vi "Main.vi"(8 "error in":errorcluster, 11 "Workers in":refnum<class "Workers.lvclass">) -> (0 "error out":errorcluster, 3 "Workers out":refnum<class "Workers.lvclass">)   [LabVIEW 2025, in "Workers.lvclass"]
doc: "The <b>Queued Message Handler</b> of the Worker that owns this VI."
uses:
  Workers.lvclass
  C:/Program Files (x86)/National Instruments/LabVIEW 2025/vi.lib/addons/_Workers/Library/Classes/Worker/Worker.lvclass
  Initialization Data.ctl
  Response Cases.ctl
  Workers.lvclass/Workers.ctl
  AnotherWorkers/AnotherWorkers.lvclass
  rql_PressGetDateTime.ctl
  rql_PressGenerateRandomNum.ctl
  rql_PressReturnRandomNum.ctl
  rql_PressReturnPasswordKey.ctl
  <vilib>/addons/_Workers/Library/Classes/Message Queue/Message Queue.lvclass
  <vilib>/addons/_Workers/Library/Classes/Worker/Worker.lvclass
  C:/Program Files (x86)/National Instruments/LabVIEW 2025/vi.lib/addons/_Workers/Library/Classes/Workers Object/Workers Object.lvclass
  C:/Users/chrismadlax/Desktop/LVSampleCode/WorkersUML/Workers/Workers/Workers.lvclass
  AnotherWorkers/rqp_GeneratePasswordKey.ctl
  C:/Users/chrismadlax/Desktop/LVSampleCode/WorkersUML/Workers/AnotherWorkers/AnotherWorkers.lvclass
panel:
  out "String 2":string
  in  "CallAnotherWorker:ReturnPasswordKEY":bool
  out "String":string
  in  "CallAnotherWorker:ReturnRandomNum":bool
  in  "CallAnotherWorker:GenerateRandomNum":bool
  in  "GetDateTime":bool
  # "Workers"
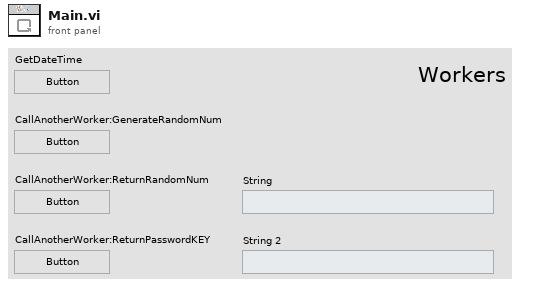
[diagram p1: front panel]
types:
  T1 = typedef "Workers.lvclass/Initialization Data.ctl" = cluster{"Response Cases":T2}
  T2 = typedef "Workers.lvclass/Response Cases.ctl" = cluster{"Placeholder - Can be deleted":string}
  T3 = typedef "Workers.lvclass/rql_PressGetDateTime.ctl" = cluster{"String":string}
  T4 = typedef "Workers.lvclass/rql_PressGenerateRandomNum.ctl" = cluster{"String":string}
  T5 = typedef "Workers.lvclass/rql_PressReturnRandomNum.ctl" = cluster{"String":string}
  T6 = typedef "AnotherWorkers.lvclass/rqp_GeneratePasswordKey.ctl" = cluster{"String":string}
  T7 = typedef "Workers.lvclass/rql_PressReturnPasswordKey.ctl" = cluster{"String":string}
  T8 = typedef "AnotherWorkers.lvclass/rwr_ReturnRandomNumber Reply.ctl" = cluster{"String":string}
  T9 = typedef "Workers.lvlib/Case Label.ctl" = string
  T10 = typedef "AnotherWorkers.lvclass/rsp_ReturnPasswordKey.ctl" = cluster{"String":string}
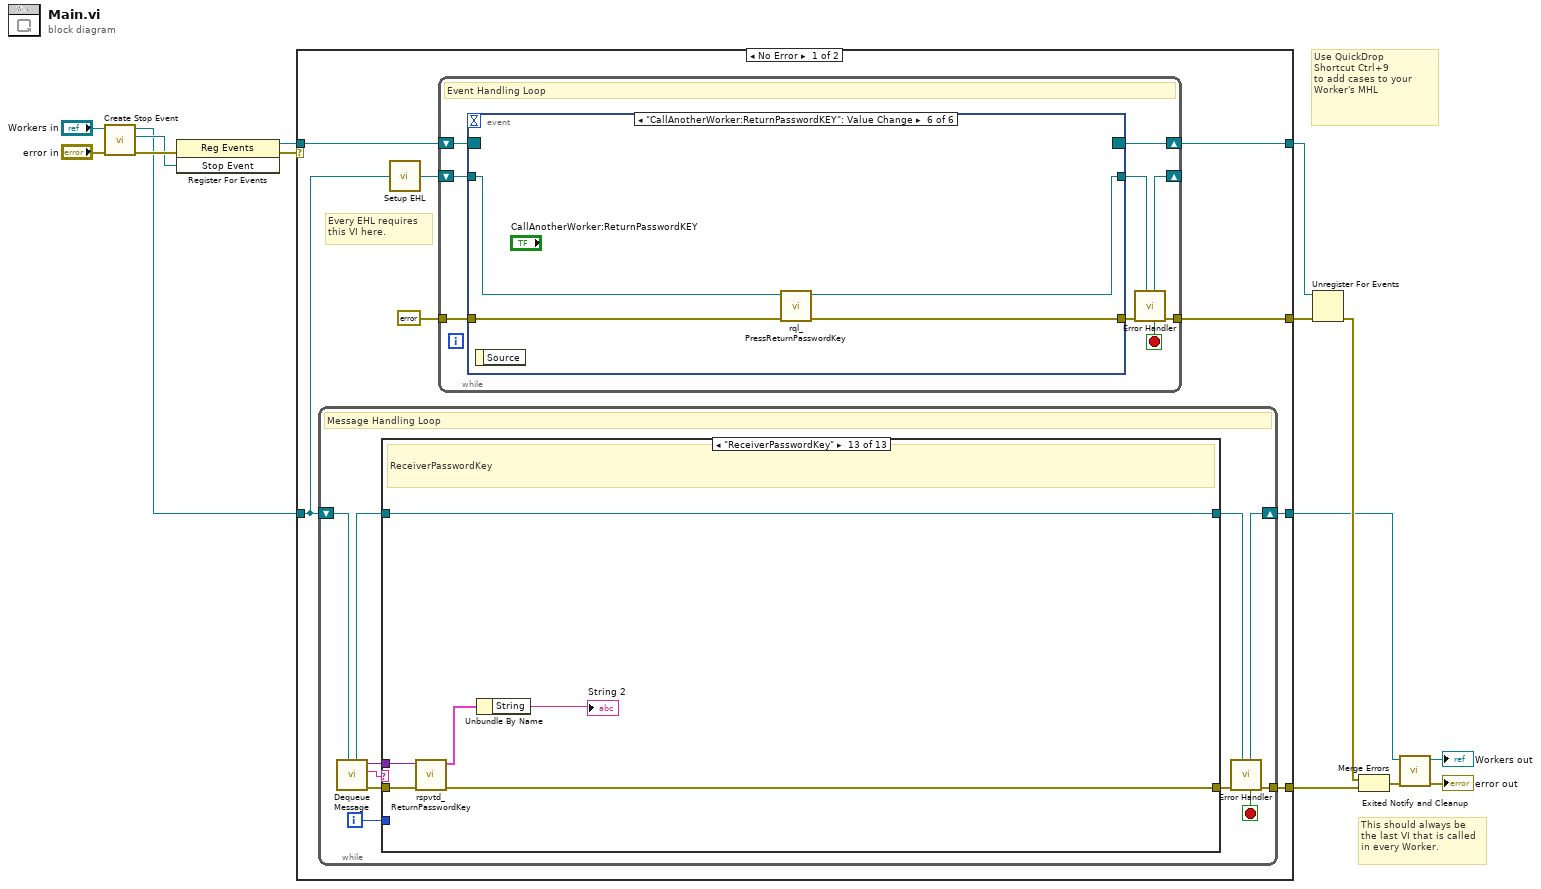
[diagram p0: block diagram]
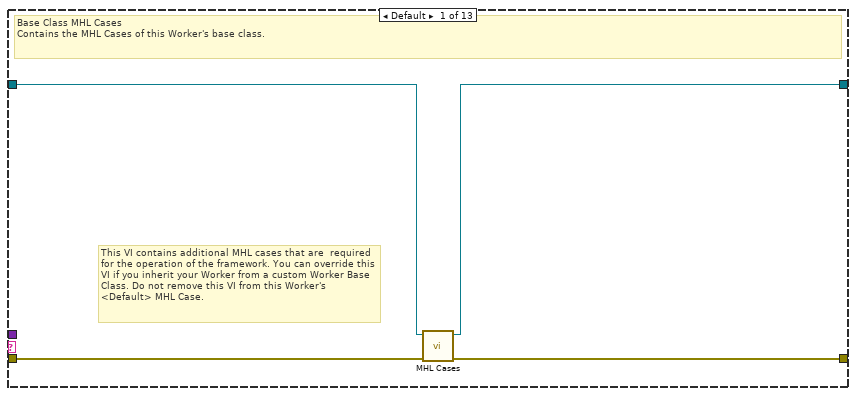
[diagram p2: hidden frame]
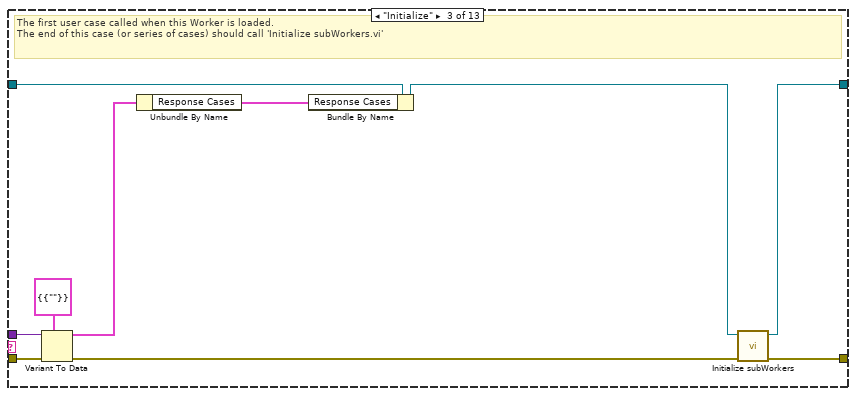
[diagram p4: hidden frame]
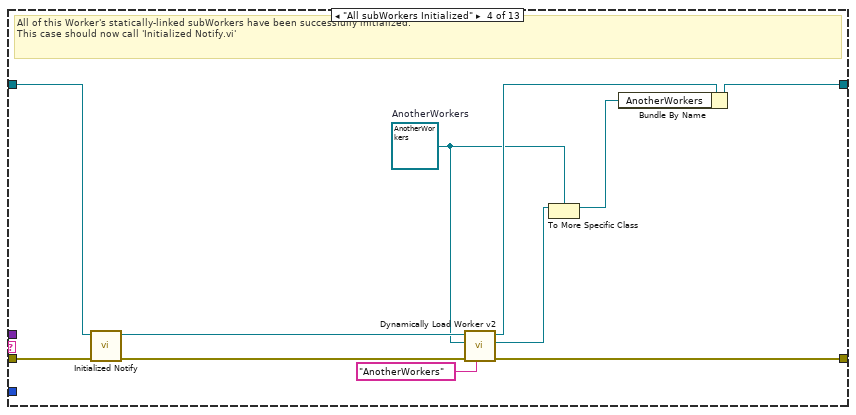
[diagram p5: hidden frame]
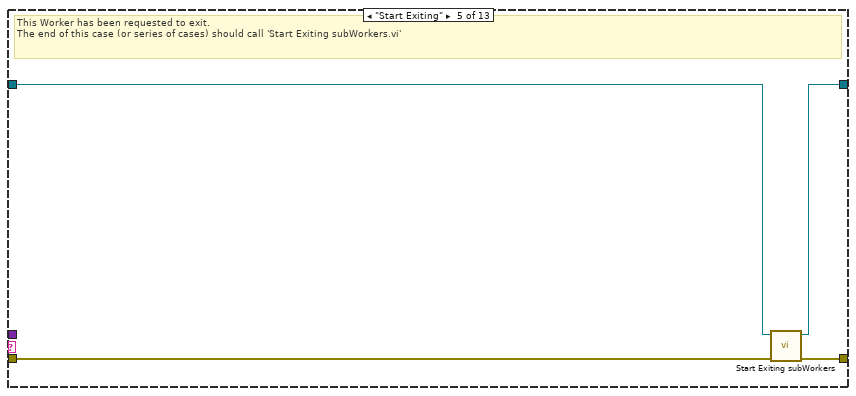
[diagram p6: hidden frame]
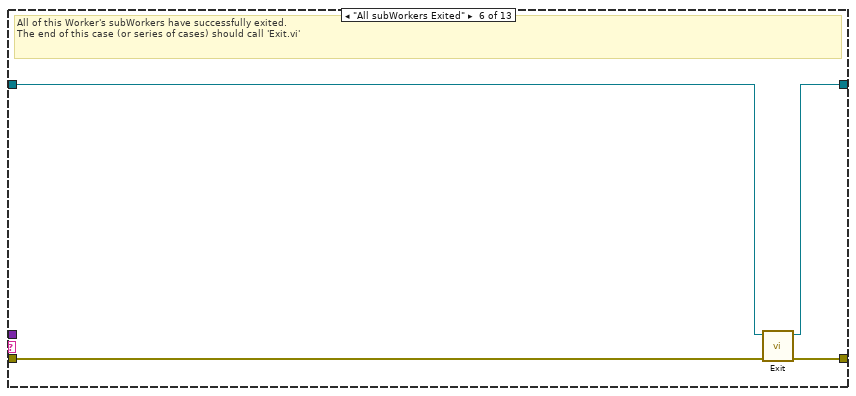
[diagram p7: hidden frame]
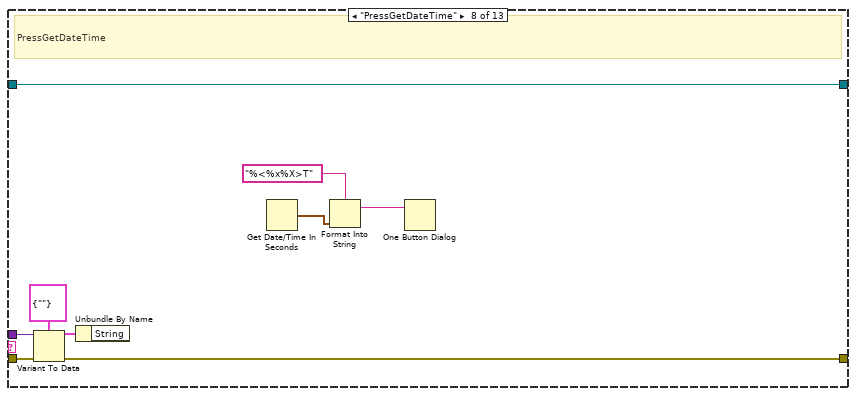
[diagram p9: hidden frame]
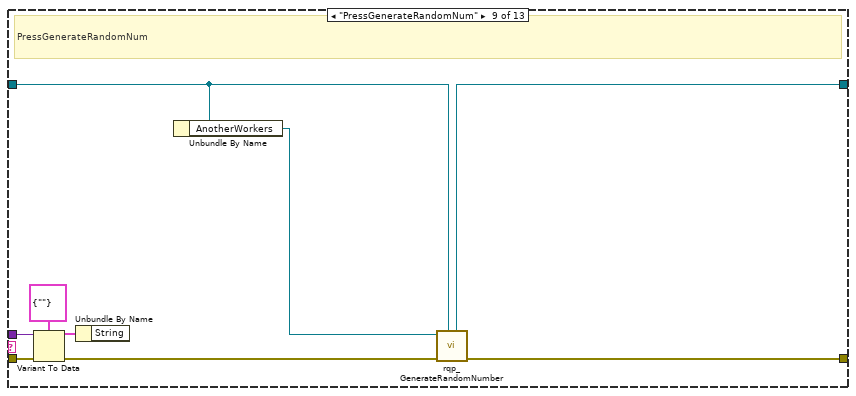
[diagram p10: hidden frame]
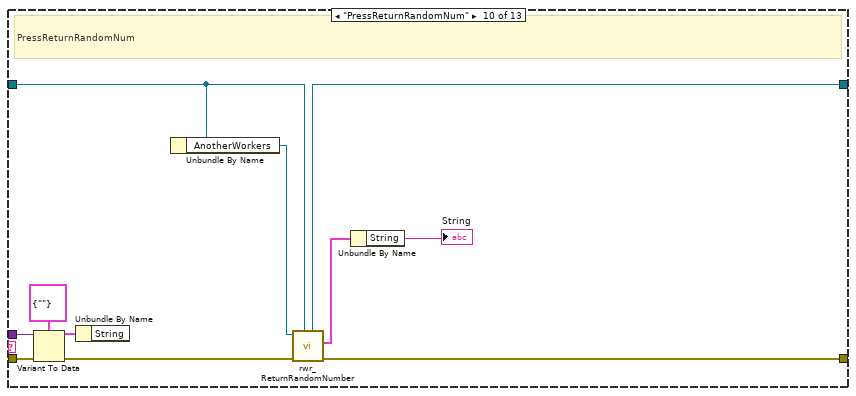
[diagram p11: hidden frame]
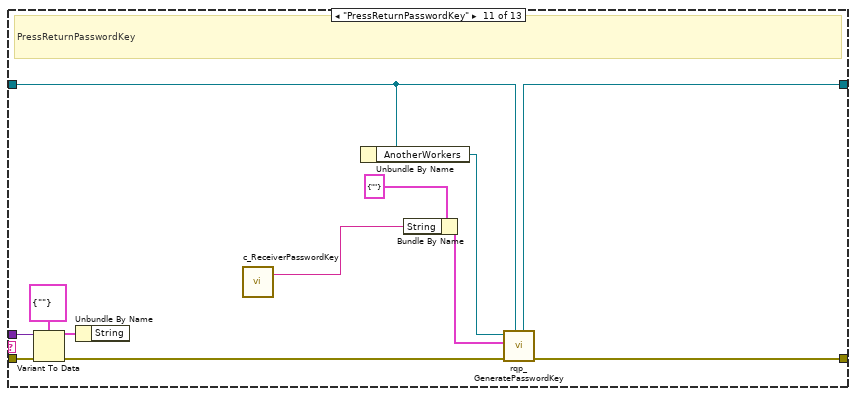
[diagram p12: hidden frame]
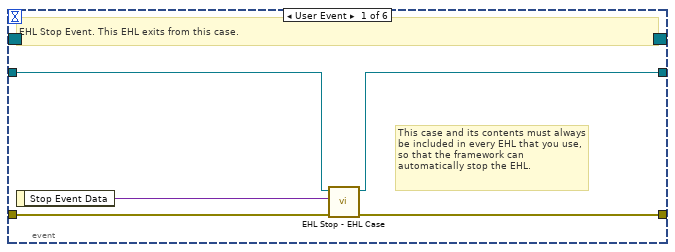
[diagram p14: hidden frame]
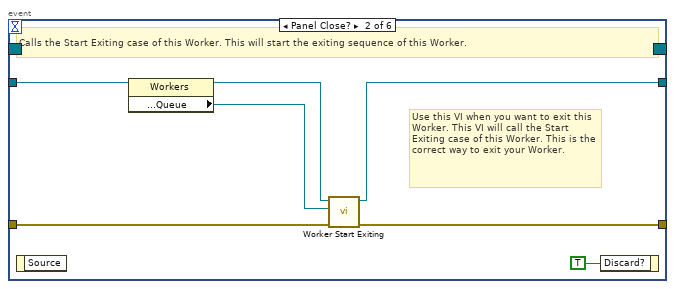
[diagram p15: hidden frame]
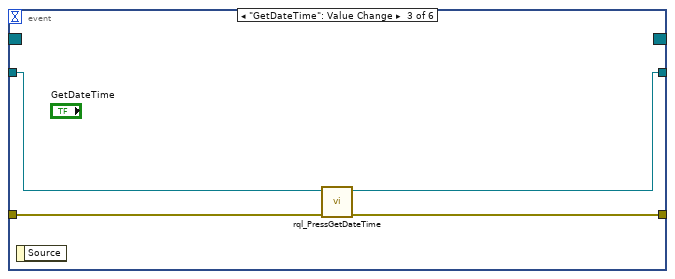
[diagram p16: hidden frame]
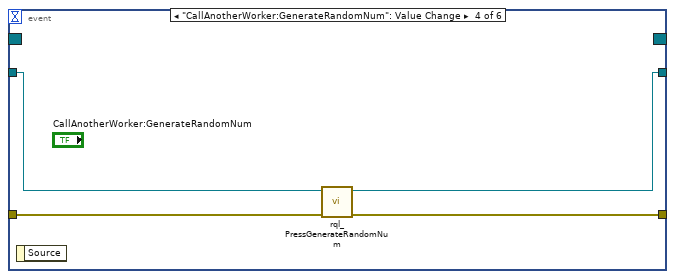
[diagram p17: hidden frame]
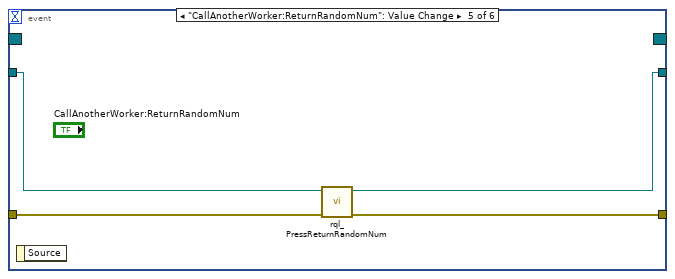
[diagram p18: hidden frame]
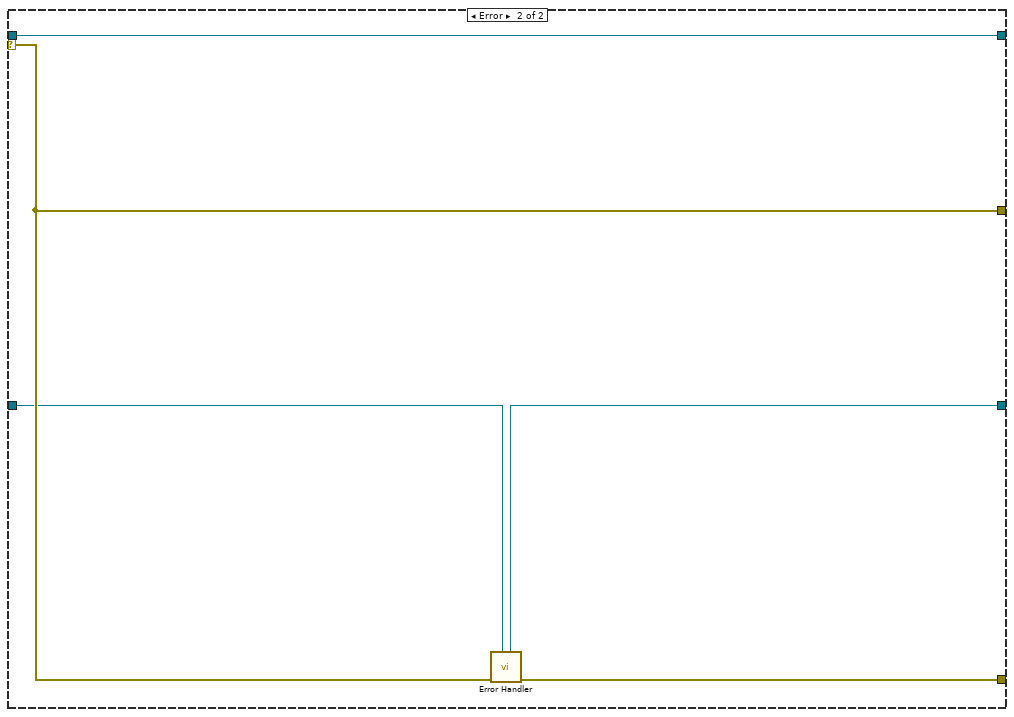
[diagram p19: hidden frame]
diagram:
  # "Use QuickDrop\nShortcut Ctrl+9\nto add cases to your\nWorker's MHL"
  # "This should always be the last VI that is called in every Worker."
  n1 = call-dynamic "Create Stop Event.vi"("error in"="error in", "Worker"="Workers in") -> ("error out"=w10:errorcluster, "Stop Event"=w7:refnum<user-event>, "Worker out"=w4:refnum<class "Workers.lvclass">)  [unwired: 7 in]
  n2 = register-events(error in=w10, w7) -> (reference out=w9:refnum<event-registration>, error out=w1:errorcluster)  [unwired: 1 in]
  n3 = case shown="No Error" w1 {
    tunnel: w4 -> [w18 w159]
    tunnel: [w16 w160] -> w8
    tunnel: w9 -> [w23 w161]
    tunnel: [w20 w162] -> w14
    tunnel: [w22 w161] -> w13
    tunnel: [w17 w158] -> w11
    selector: w1 -> [_ w162]
    frame No Error {
      # "Every EHL requires\nthis VI here."
      n4 = while {
        shift-right: [w32] -> w17
        shift-left: w18 -> [w34]
        tunnel: [w33] -> w16
        i -> [w25]
        stop <- w26 stop-if-true
        # "Message Handling Loop"
        n5 = call-dynamic "Dequeue Message.vi"("Worker"=w34) -> ("error out"=w31:errorcluster, "Case out"=w27:string, "Data out"=w24:variant, "Worker out"=w29:refnum<class "Workers.lvclass">)  [unwired: 6 in, 1 out]
        n6 = case "Worker MHL Case Structure (DO NOT CHANGE LABEL NAME)" shown="\"ReceiverPasswordKey\"" w27 {
          tunnel: w31 -> [w38 w39 w48 w60 w62 w69 w71 w79 w89 w100 w112 w114 w120]
          tunnel: [w37 w39 w50 w58 w65 w68 w71 w78 w84 w95 w107 w114 w118] -> w30
          tunnel: w29 -> [w36 w40 w47 w61 w63 w67 w70 w80 w82 w93 w105 w113 w119]
          tunnel: [w35 w40 w49 w54 w64 w66 w70 w80 w83 w94 w106 w113 w119] -> w28
          tunnel: w25 -> [_ _ _ _ _ _ _ _ _ _ _ _ _]
          tunnel: w24 -> [_ _ w45 _ _ _ _ w76 w86 w97 w109 _ w117]
          frame Default {
            # "This VI contains additional MHL cases that are  required for the operation of the framework. You can override this VI if you inherit your Worker from a custom Worker Base Class. Do not remove this VI from this Worker's <Default> MHL Case."
            # "Base Class MHL Cases\nContains the MHL Cases of this Worker's base class."
            n7 = call-dynamic "MHL Cases.vi"("error in"=w38, "Worker in"=w36) -> ("error out"=w37:errorcluster, "Worker out"=w35:refnum<class "Workers.lvclass">)  [unwired: 8 in]
          }
          frame "------------ FRAMEWORK CASES -----------" {
            # "Start of Workers Framework Cases"
          }
          frame "Initialize" {
            # "The first user case called when this Worker is loaded.\nThe end of this case (or series of cases) should call 'Initialize subWorkers.vi'"
            n8 = Variant To Data(error in=w48, type=T1 {"Response Cases"={"Placeholder - Can be deleted"=""}} ("Initialization Data"), Variant=w45) -> (data=w43:T1, error out=w46:errorcluster)
            n9 = Unbundle By Name(w43) -> ("Response Cases"=w42:T2)
            n10 = Bundle By Name(cluster=w47, "Response Cases"=w42) -> (w44:refnum<class "Workers.lvclass">)
            n11 = call-dynamic "Initialize subWorkers.vi"("error in"=w46, "Worker"=w44) -> ("error out"=w50:errorcluster, "dup Worker out"=w49:refnum<class "Workers.lvclass">)  [unwired: 8 in]
          }
          frame "All subWorkers Initialized" {
            w51 = refnum<class "AnotherWorkers.lvclass"> refnum  # AnotherWorkers
            # "All of this Worker's statically-linked subWorkers have been successfully initialized.\nThis case should now call 'Initialized Notify.vi'"
            n12 = call-dynamic "Initialized Notify.vi"("error in"=w60, "Worker"=w61) -> ("error out"=w59:errorcluster, "dup Worker out"=w57:refnum<class "Workers.lvclass">)  [unwired: 8 in]
            n13 = call <vilib>:"Dynamically Load Worker v2.vi"("Worker Alias"="AnotherWorkers", "error in"=w59, "Worker to Dynamically Load"=w51, "Worker"=w57) -> ("error out"=w58:errorcluster, "Dynamically Loaded Worker out"=w52:refnum<class "Worker.lvclass">, "dup Worker out"=w56:refnum<class "Workers.lvclass">)  [unwired: 5 in]
            n14 = To More Specific Class(target class=w51, reference=w52) -> (specific class reference=w53:refnum<class "AnotherWorkers.lvclass">)  [unwired: 1 in, 1 out]
            n15 = Bundle By Name(cluster=w56, "AnotherWorkers"=w53) -> (w54:refnum<class "Workers.lvclass">)
          }
          frame "Start Exiting" {
            # "This Worker has been requested to exit. \nThe end of this case (or series of cases) should call 'Start Exiting subWorkers.vi'"
            n16 = call-dynamic "Start Exiting subWorkers.vi"("error_in"=w62, "Worker"=w63) -> ("error out"=w65:errorcluster, "dup Worker out"=w64:refnum<class "Workers.lvclass">)  [unwired: 8 in]
          }
          frame "All subWorkers Exited" {
            # "All of this Worker's subWorkers have successfully exited. \nThe end of this case (or series of cases) should call 'Exit.vi'"
            n17 = call-dynamic "Exit.vi"("error_in"=w69, "Worker"=w67) -> ("error out"=w68:errorcluster, "dup Worker out"=w66:refnum<class "Workers.lvclass">)  [unwired: 8 in]
          }
          frame "------------- LOCAL API CASES -------------" {
            # "Start of Workers Local API Cases"
          }
          frame "PressGetDateTime" {
            # "PressGetDateTime"
            n18 = Variant To Data(error in=w79, type=T3 {"String"=""} ("Data"), Variant=w76) -> (data=w75:T3, error out=w78:errorcluster)
            n19 = Unbundle By Name(w75) -> ()  [unwired: 1 out]
            n20 = Get Date/Time In Seconds() -> (seconds since 1Jan1904=w74:timestamp)
            n21 = Format Into String(format string="%<%x%X>T", w74) -> (resulting string=w72:string)  [unwired: 2 in, 1 out]
            n22 = One Button Dialog(message=w72) -> ()  [unwired: 1 in, 1 out]
          }
          frame "PressGenerateRandomNum" {
            # "PressGenerateRandomNum"
            n23 = Variant To Data(error in=w89, type=T4 {"String"=""} ("Data"), Variant=w86) -> (data=w85:T4, error out=w88:errorcluster)
            n24 = Unbundle By Name(w85) -> ()  [unwired: 1 out]
            n25 = Unbundle By Name(w82) -> ("AnotherWorkers"=w81:refnum<class "AnotherWorkers.lvclass">)
            n26 = call "rqp_GenerateRandomNumber.vi"("Caller in"=w82, "error in"=w88, "AnotherWorkers in"=w81) -> ("error out"=w84:errorcluster, "dup Caller out"=w83:refnum<class "Workers.lvclass">)  [unwired: 6 in, 1 out]
          }
          frame "PressReturnRandomNum" {
            # "PressReturnRandomNum"
            n27 = Variant To Data(error in=w100, type=T5 {"String"=""} ("Data"), Variant=w97) -> (data=w96:T5, error out=w99:errorcluster)
            n28 = Unbundle By Name(w96) -> ()  [unwired: 1 out]
            n29 = Unbundle By Name(w93) -> ("AnotherWorkers"=w92:refnum<class "AnotherWorkers.lvclass">)
            n30 = call "rwr_ReturnRandomNumber.vi"("Caller in"=w93, "error in"=w99, "AnotherWorkers in"=w92) -> ("error out"=w95:errorcluster, "Reply Data out"=w91:T8, "dup Caller out"=w94:refnum<class "Workers.lvclass">)  [unwired: 5 in, 1 out]
            n31 = Unbundle By Name(w91) -> ("String"=→"String":string)
          }
          frame "PressReturnPasswordKey" {
            # "PressReturnPasswordKey"
            n32 = Variant To Data(error in=w112, type=T7 {"String"=""} ("Data"), Variant=w109) -> (data=w108:T7, error out=w111:errorcluster)
            n33 = Unbundle By Name(w108) -> ()  [unwired: 1 out]
            n34 = call "c_ReceiverPasswordKey.vi"() -> ("Case Label"=w101:T9)  [unwired: 1 in]
            n35 = Unbundle By Name(w105) -> ("AnotherWorkers"=w104:refnum<class "AnotherWorkers.lvclass">)
            n36 = Bundle By Name(cluster=T6 {"String"=""} ("Data in"), "String"=w101) -> (w102:T6)
            n37 = call "rqp_GeneratePasswordKey.vi"("Caller in"=w105, "error in"=w111, "Data in"=w102, "AnotherWorkers in"=w104) -> ("error out"=w107:errorcluster, "dup Caller out"=w106:refnum<class "Workers.lvclass">)  [unwired: 5 in, 1 out]
          }
          frame "------------- RESPONSE CASES --------------" {
            # "Start of Workers Response Cases"
          }
          frame "ReceiverPasswordKey" {
            # "ReceiverPasswordKey"
            n38 = call "rspvtd_ReturnPasswordKey.vi"("error in"=w120, "Data in"=w117) -> ("error out"=w118:errorcluster, "Data out"=w116:T10)  [unwired: 8 in]
            n39 = Unbundle By Name(w116) -> ("String"=→"String 2":string)
          }
        }
        n40 = call-dynamic "Error Handler.vi"("Worker"=w28, "error_in"=w30) -> ("error out"=w33:errorcluster, "Stop Loop"=w26:bool, "Worker out"=w32:refnum<class "Workers.lvclass">)  [unwired: 7 in]
      }
      n41 = call-dynamic "Setup EHL.vi"("Worker"=w18) -> ("Worker out"=w19:refnum<class "Workers.lvclass">)  [unwired: 14 in]
      n42 = while "Event Handling Loop" {
        shift-right: [w129] -> w22
        shift-left: w23 -> [w128]
        tunnel: [w124] -> w20
        tunnel: errorcluster {"status"=FALSE, "code"=0, "source"=""} ("error constant") -> [w126]
        shift-right: [w122] -> _
        shift-left: w19 -> [w127]
        stop <- w121 stop-if-true
        # "Event Handling Loop"
        n43 = event shown="[5] \"CallAnotherWorker:ReturnPasswordKEY\": Value Change" {
          selector: w128 -> [_ _ _ _ _ _]
          dyn-events: [_ _ _ _ _ _] -> w129
          timeout: _ -> [_ _ _ _ _ _]
          tunnel: [w133 w140 w144 w148 w152 w156] -> w125
          tunnel: w126 -> [w134 w139 w145 w149 w153 w157]
          tunnel: w127 -> [w132 w138 w143 w147 w151 w155]
          tunnel: [w131 w137 w142 w146 w150 w154] -> w123
          event User Event {
            # "This case and its contents must always be included in every EHL that you use, so that the framework can automatically stop the EHL."
            # "EHL Stop Event. This EHL exits from this case."
            n44 = event-data() -> ("Stop Event Data"=w130:variant)  [unwired: 1 in]
            n45 = call-dynamic "EHL Stop - EHL Case.vi"("error in"=w134, "Stop Event Data"=w130, "Worker"=w132) -> ("error out"=w133:errorcluster, "Worker out"=w131:refnum<class "Workers.lvclass">)  [unwired: 7 in]
          }
          event Panel Close? {
            # "Use this VI when you want to exit this Worker. This VI will call the Start Exiting case of this Worker. This is the correct way to exit your Worker."
            # "Calls the Start Exiting case of this Worker. This will start the exiting sequence of this Worker."
            n46 = event-data() -> ()  [unwired: 1 in, 1 out]
            n47 = property class="Workers"(reference=w138) -> (reference out=w136:refnum<class "Workers.lvclass">, "Accessors:Read:Public API:Queue"=w135:refnum<class "Message Queue.lvclass">)  [unwired: 1 in, 1 out]
            n48 = call-dynamic "Worker Start Exiting.vi"("error_in"=w139, "Message Queue"=w135, "Worker"=w136) -> ("error out"=w140:errorcluster, "dup Worker out"=w137:refnum<class "Workers.lvclass">)  [unwired: 7 in]
            n49 = event-data("Discard?"=TRUE) -> ()  [unwired: 1 in, 1 out]
          }
          event "GetDateTime": Value Change {
            n50 = event-data() -> ()  [unwired: 1 in, 1 out]
            n51 = call "rql_PressGetDateTime.vi"("error in"=w145, "Workers in"=w143) -> ("error out"=w144:errorcluster, "dup Workers out"=w142:refnum<class "Workers.lvclass">)  [unwired: 8 in]
          }
          event "CallAnotherWorker:GenerateRandomNum": Value Change {
            n52 = event-data() -> ()  [unwired: 1 in, 1 out]
            n53 = call "rql_PressGenerateRandomNum.vi"("error in"=w149, "Workers in"=w147) -> ("error out"=w148:errorcluster, "dup Workers out"=w146:refnum<class "Workers.lvclass">)  [unwired: 8 in]
          }
          event "CallAnotherWorker:ReturnRandomNum": Value Change {
            n54 = event-data() -> ()  [unwired: 1 in, 1 out]
            n55 = call "rql_PressReturnRandomNum.vi"("error in"=w153, "Workers in"=w151) -> ("error out"=w152:errorcluster, "dup Workers out"=w150:refnum<class "Workers.lvclass">)  [unwired: 8 in]
          }
          event "CallAnotherWorker:ReturnPasswordKEY": Value Change {
            n56 = event-data() -> ()  [unwired: 1 in, 1 out]
            n57 = call "rql_PressReturnPasswordKey.vi"("error in"=w157, "Workers in"=w155) -> ("error out"=w156:errorcluster, "dup Workers out"=w154:refnum<class "Workers.lvclass">)  [unwired: 8 in]
          }
        }
        n58 = call-dynamic "Error Handler.vi"("Worker"=w123, "error_in"=w125) -> ("error out"=w124:errorcluster, "Stop Loop"=w121:bool, "Worker out"=w122:refnum<class "Workers.lvclass">)  [unwired: 7 in]
      }
    }
    frame Error {
      n59 = call-dynamic "Error Handler.vi"("Worker"=w159, "error_in"=w162) -> ("error out"=w160:errorcluster, "Worker out"=w158:refnum<class "Workers.lvclass">)  [unwired: 7 in, 1 out]
    }
  }
  n60 = Unregister For Events(event registration refnum=w13, error in=w14) -> (error out=w15:errorcluster)
  n61 = Merge Errors(w15, w8) -> (w12:errorcluster)
  n62 = call-dynamic "Exited Notify and Cleanup.vi"("error_in"=w12, "Worker"=w11) -> ("error out"=→"error out":errorcluster, "dup Worker out"=→"Workers out":refnum<class "Workers.lvclass">)  [unwired: 8 in]
